vi "JSONtext Pretty Print.vi"(11 "JSON":string) -> (2 "Value String":string, 3 "Boolean":bool)   [LabVIEW 2015]
uses:
  JSONtext.lvlib
panel:
  out "String":string
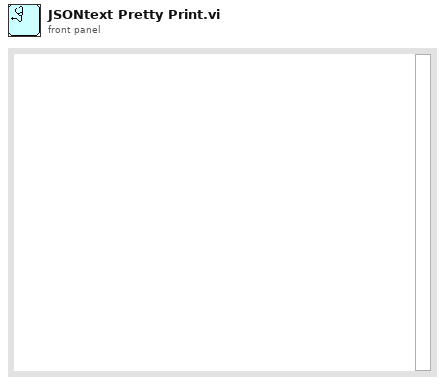
[diagram p1: front panel]
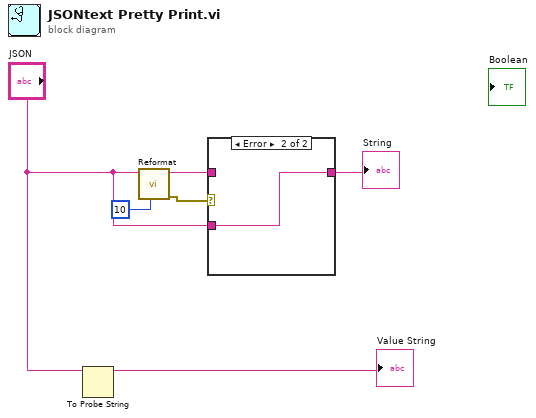
[diagram p0: block diagram]
diagram:
  n1 = To Probe String(7:"JSON") -> (3:→"Value String":string)  [unwired: 2 in, 1 out]
  n2 = call "Reformat.vi"("Pretty Print Levels"=10, "Input String"="JSON") -> ("error out"=w5:errorcluster, "<JSON>First JSON Value"=w4:string)  [unwired: 6 in, 2 out]
  n3 = case shown="Error" w5 {
    tunnel: [w7 w8] -> w3
    tunnel: w4 -> [w7 _]
    tunnel: "JSON" -> [_ w8]
    frame No Error {
    }
    frame Error {
    }
  }
  "String" <- w3
